vi "Verify Baseline Directory.vi"(8 "error in":errorcluster, 10 "Baseline Directory":path, 11 "Peer Review in":refnum<class "Peer Review.lvclass">) -> (0 "error out":errorcluster, 3 "Peer Review out":refnum<class "Peer Review.lvclass">)   [LabVIEW 2020, in "Peer Review.lvclass"]
uses:
  Peer Review.lvclass
  Peer Review.lvclass/Peer Review.ctl
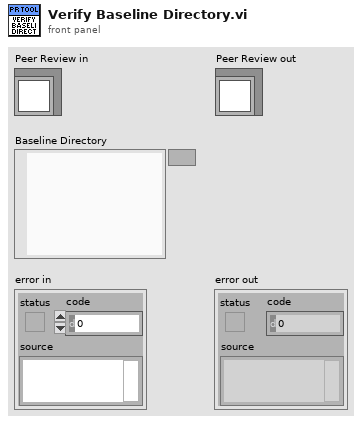
[diagram p1: front panel]
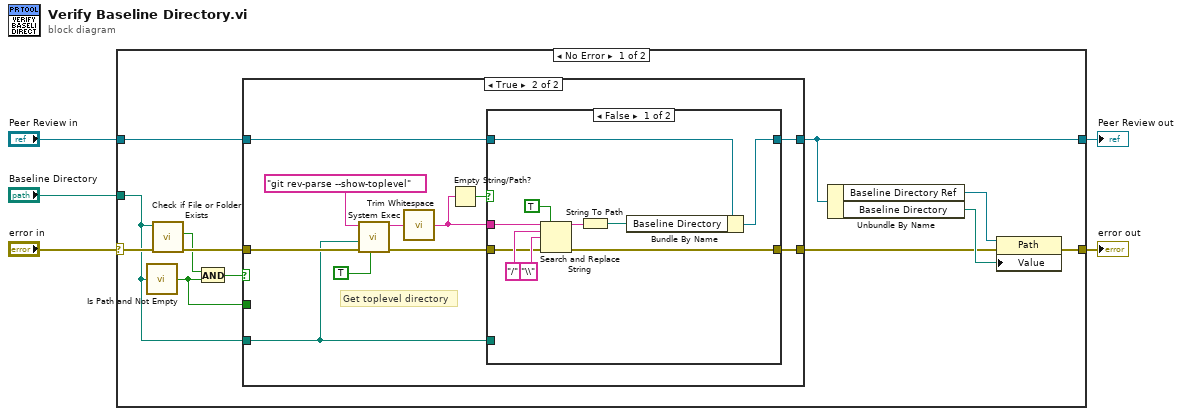
[diagram p0: block diagram]
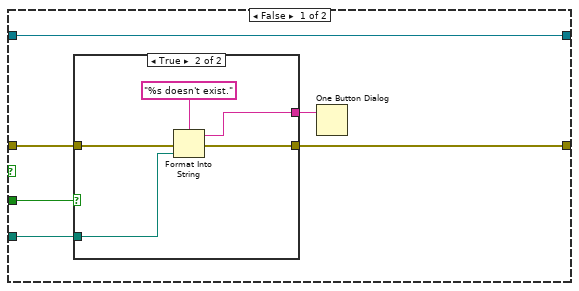
[diagram p2: hidden frame]
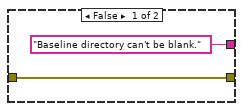
[diagram p3: hidden frame]
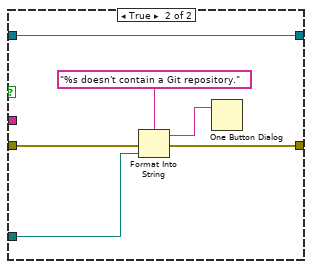
[diagram p4: hidden frame]
diagram:
  n1 = case shown="No Error" "error in" {
    selector: "error in" -> [w16 w59]
    tunnel: [w7 w59] -> w4
    tunnel: [w6 w58] -> w2
    tunnel: "Peer Review in" -> [w17 w58]
    tunnel: "Baseline Directory" -> [w12 _]
    frame No Error {
      n2 = call <vilib>:"Is Path and Not Empty.vi"("path"=w12) -> ("Is Path and Not Empty?"=w11:bool)  [unwired: 4 in]
      n3 = call <vilib>:"Check if File or Folder Exists.vi"("error in (no error)"=w16, "path"=w12) -> ("error out"=w15:errorcluster, "file or folder exists?"=w14:bool)  [unwired: 7 in, 1 out]
      n4 = And(x=w14, y=w11) -> (x .and. y?=w13:bool)
      n5 = case shown="True" w13 {
        tunnel: w17 -> [w21 w38]
        tunnel: [w18 w31] -> w8
        tunnel: [w21 w32] -> w6
        tunnel: w15 -> [w23 w35]
        tunnel: w12 -> [w22 w34]
        tunnel: w11 -> [w19 _]
        frame False {
          n6 = case shown="True" w19 {
            tunnel: w23 -> [w25 w29]
            tunnel: w22 -> [_ w28]
            tunnel: [w25 w27] -> w18
            tunnel: ["Baseline directory can't be blank." ("error message (\"\")") w26] -> w20
            frame False {
            }
            frame True {
              n7 = Format Into String(format string="%s doesn't exist." ("error message (\"\")"), error in=w29, w28) -> (resulting string=w26:string, error out=w27:errorcluster)  [unwired: 1 in]
            }
          }
          n8 = One Button Dialog(message=w20) -> ()  [unwired: 1 in, 1 out]
        }
        frame True {
          # "Get toplevel directory"
          n9 = call <vilib>:"System Exec.vi"("run minimized? (F)"=TRUE, "error in (no error)"=w35, "working directory"=w34, "command line"="git rev-parse --show-toplevel" ("String 2")) -> ("error out"=w37:errorcluster, "standard output"=w41:string)  [unwired: 4 in, 2 out]
          n10 = call <vilib>:"Trim Whitespace.vi"("string"=w41) -> ("trimmed string"=w33:string)  [unwired: 1 in]
          n11 = Empty String/Path?(string/path=w33) -> (empty?=w36:bool)
          n12 = case shown="False" w36 {
            tunnel: w38 -> [w45 w53]
            tunnel: w37 -> [w46 w57]
            tunnel: [w42 w52] -> w31
            tunnel: [w43 w53] -> w32
            tunnel: w33 -> [w47 _]
            tunnel: w34 -> [_ w56]
            frame False {
              n13 = Search and Replace String(replace all?=TRUE ("replace all? (F)"), input string=w47, search string="/", replace string="\\" ("replace string (\"\")"), error in=w46) -> (result string=w51:string, error out=w42:errorcluster)  [unwired: 3 in, 2 out]
              n14 = String To Path(string=w51) -> (path=w44:path)
              n15 = Bundle By Name(cluster=w45, "Baseline Directory"=w44) -> (w43:refnum<class "Peer Review.lvclass">)
            }
            frame True {
              n16 = Format Into String(format string="%s doesn't contain a Git repository." ("error message (\"\")"), error in=w57, w56) -> (resulting string=w54:string, error out=w52:errorcluster)  [unwired: 1 in]
              n17 = One Button Dialog(message=w54) -> ()  [unwired: 1 in, 1 out]
            }
          }
        }
      }
      n18 = Unbundle By Name(w6) -> ("Baseline Directory Ref"=w10:refnum<vi>, "Baseline Directory"=w9:path)
      n19 = property class="Path"(reference=w10, error in=w8, "Value"=w9) -> (error out=w7:errorcluster)  [unwired: 1 out]
    }
    frame Error {
    }
  }
  "error out" <- w4
  "Peer Review out" <- w2
